vi "Init.vi"(6 "Init Implementations":T2, 7 "App Version":string, 8 "error in (no error)":errorcluster, 9 "Minimum Event Level (Info)":T1=enum."Info", 10 "Node":refnum<class "Node Config.lvclass">) -> (0 "error out":errorcluster, 3 "Vecto out":refnum<class "Vecto.lvclass">)   [LabVIEW 2020, in "Vecto.lvlib" / "Vecto.lvclass"]
uses:
  Vecto.lvclass
  Node Config/Node Config.lvclass
  Init Implementations.ctl
  EventLogHandler/EventLogHandler.lvclass
  Event Level.ctl
  Vecto.lvclass/Vecto.ctl
  EventLoggingService/EventLoggingService.lvclass
  Vecto.lvlib
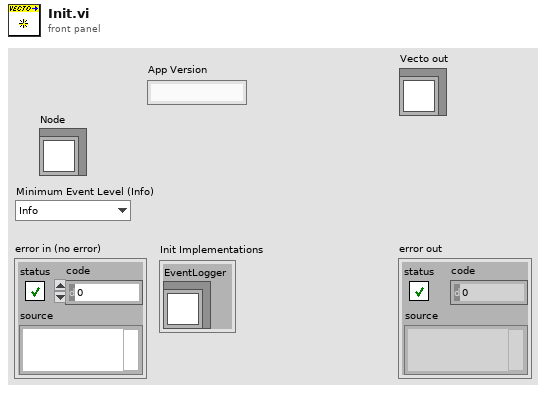
[diagram p1: front panel]
types:
  T1 = typedef "Vecto.lvlib/Event Level.ctl" = enum16{"Debug", "Info", "Warning", "Error"}
  T2 = typedef "Vecto.lvlib/Init Implementations.ctl" = cluster{"EventLogger":refnum<class "EventLogHandler.lvclass">}
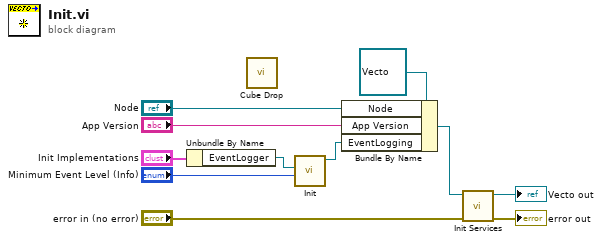
[diagram p0: block diagram]
diagram:
  n1 = Unbundle By Name("Init Implementations") -> ("EventLogger"=w2:refnum<class "EventLogHandler.lvclass">)
  n2 = call "Cube Drop.vi"() -> ()  [unwired: 12 in]
  n3 = call "Init.vi"("Minimum Event Level"="Minimum Event Level (Info)", "EventLogger"=w2) -> ("EventLoggingService out"=w1:refnum<class "EventLoggingService.lvclass">)  [unwired: 8 in, 1 out]
  n4 = Bundle By Name(cluster=refnum<class "Vecto.lvclass"> refnum ("Vecto in"), "Node"="Node", "App Version"="App Version", "EventLogging"=w1) -> (w9:refnum<class "Vecto.lvclass">)
  n5 = call "Init Services.vi"("error in (no error)"="error in (no error)", "Vecto in"=w9) -> ("error out"=→"error out":errorcluster, "Vecto out"=→"Vecto out":refnum<class "Vecto.lvclass">)  [unwired: 8 in]
